vi "Begin.vi"(11 "Image Size":T1=enum."160x120") -> (0 "error out":errorcluster)   [LabVIEW 2012]
doc: "Called before other user functions, this VI is expected to open initial I/O refnums, load in file data, and do all program initialization. Notice that the <B>error out</B> terminal is simply used for data flow. Wiring it to other structures or subVIs ensures that this VI runs first."
uses:
  <vilib>/Rock Robotics/WPI/Camera/WPI_CameraImageSize.ctl
  <vilib>/Rock Robotics/WPI/Camera/WPI_CameraWhite Balance Values.ctl
  <vilib>/Rock Robotics/WPI/Camera/WPI_CameraExposure Values.ctl
  <vilib>/Rock Robotics/WPI/Camera/WPI_CameraFrameRate.ctl
  <vilib>/Rock Robotics/WPI/DriverStation/WPI_DriverStationRobotMode2.ctl
  <vilib>/Rock Robotics/SystemInterfaces/DIO/FPGA_DIOPWMChannel.ctl
  <vilib>/Rock Robotics/WPI/Joystick/WPI_JoystickDeviceEnum.ctl
  <vilib>/Rock Robotics/SystemInterfaces/Typedef/FPGA_TypedefDigitalModule.ctl
  Robot Global Data.vi
  <vilib>/Rock Robotics/WPI/MotorControl/WPI_MotorControlOpen Victor.vi
  <vilib>/Rock Robotics/SystemInterfaces/DIO/FPGA_DIOChannel.ctl
  <vilib>/Rock Robotics/SystemInterfaces/AI/FPGA_AIGyroChannel.ctl
  <vilib>/Rock Robotics/WPI/Relay/WPI_RelayDirection.ctl
  <vilib>/Rock Robotics/SystemInterfaces/DIO/FPGA_DIORelayChannel.ctl
  <vilib>/Rock Robotics/SystemInterfaces/AI/FPGA_AIChannel.ctl
  <vilib>/Rock Robotics/WPI/MotorControl/WPI_MotorControlOpen Jaguar.vi
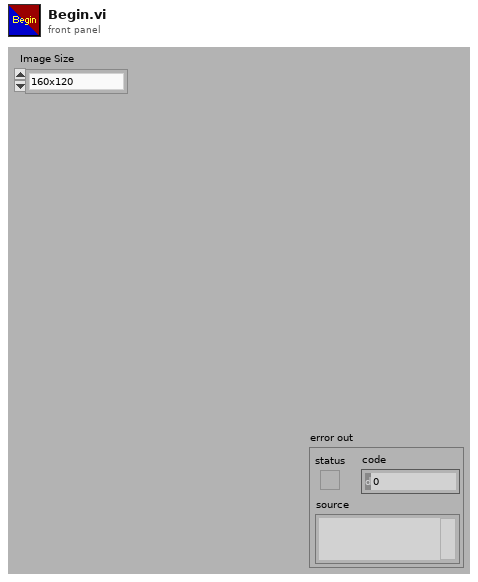
[diagram p1: front panel]
types:
  T1 = typedef "WPI_CameraImageSize.ctl" = enum16{"640x480", "320x240", "160x120"}
  T2 = typedef "FPGA_TypedefDigitalModule.ctl" = enum16{"Digital Module 1", "Digital Module 2"}
  T3 = typedef "FPGA_DIOPWMChannel.ctl" = enum8{"PWM 1", "PWM 2", "PWM 3", "PWM 4", "PWM 5", "PWM 6", "PWM 7", "PWM 8", "PWM 9", "PWM 10", "Invalid"}
  T4 = typedef "WPI_JoystickDeviceEnum.ctl" = enum16{"USB 1", "USB 2", "USB 3", "USB 4", "Kinect 1", "Kinect 2"}
  T5 = typedef "WPI_DriverStationRobotMode2.ctl" = enum16{"Autonomous Disabled", "Autonomous Enabled", "Teleop Disabled", "Teleop Enabled", "Timeout", "Finish", "Test Disabled", "Test Enabled"}
  T6 = typedef "WPI_CameraFrameRate.ctl" = u32
  T7 = typedef "WPI_CameraExposure Values.ctl" = enum16{"Auto", "Flicker-free 50 Hz", "Flicker-free 60 Hz", "Hold current"}
  T8 = typedef "WPI_CameraWhite Balance Values.ctl" = enum16{"Auto", "Fixed indoor", "Fixed outdoor 1", "Fixed outdoor 2", "Fixed fluorescent 1", "Fixed fluorescent 2", "Hold current"}
  T9 = typedef "WPI_CameraDevRef.ctl" = cluster{"Camera Address":string, "CameraStatus":errorcluster, "Acquire Image Notifier":refnum<notifier>}
  T10 = typedef "WPI_MotorControlDeviceRef.ctl" = cluster{"DeviceStatus":errorcluster, "Type":enum16{"PWM", "CAN"}, "PWM":cluster{"Digital Module":T2, "PWM Channel":T3, "DeadBand":T11}, "CAN":cluster{"Device Number":u8, "Control Mode":T12, "Semaphore":T13, "Max Vout":dbl}, "Invert":bool, "TransformRef":T14, "InvTransformRef":T14}
  T11 = typedef "WPI_PWMDeadband.ctl" = cluster{"Name":string, "maxPositivePwm":i32, "minPositivePwm":i32, "centerPwm":i32, "maxNegativePwm":i32, "minNegativePwm":i32, "angularRange":u16}
  T12 = typedef "WPI_CANJaguar_ControlMode.ctl" = enum8{"Percent VBus", "Current", "Speed", "Position", "Voltage"}
  T13 = typedef "Semaphore RefNum" = refnum<k1>
  T14 = typedef "WPI_PWMTransform_ConPane.ctl" = refnum<vi>
  T15 = typedef "WPI_JoystickDevRef.ctl" = cluster{"Device":T4}
  T16 = typedef "WPI_ServoDeviceRef.ctl" = cluster{"DeviceStatus":errorcluster, "Digital Module":T2, "PWM Channel":T3, "DeadBand":T11}
  T17 = typedef "FPGA_DIORelayChannel.ctl" = enum8{"Relay 1", "Relay 2", "Relay 3", "Relay 4", "Relay 5", "Relay 6", "Relay 7", "Relay 8", "Invalid"}
  T18 = typedef "WPI_RelayDirection.ctl" = enum16{"Both directions", "Forward only", "Reverse only"}
  T19 = typedef "WPI_RelayDevRef.ctl" = cluster{"DevStatus":errorcluster, "Relay Channel":T17, "Digital Module":T2, "Relay Direction":T18}
  T20 = typedef "FPGA_AIGyroChannel.ctl" = enum8{"AI 1", "AI 2", "Invalid"}
  T21 = typedef "FPGA_DIOChannel.ctl" = enum8{"DIO 1", "DIO 2", "DIO 3", "DIO 4", "DIO 5", "DIO 6", "DIO 7", "DIO 8", "DIO 9", "DIO 10", "DIO 11", "DIO 12", "DIO 13", "DIO 14", "Invalid"}
  T22 = typedef "FPGA_AIChannel.ctl" = enum8{"AI 1", "AI 2", "AI 3", "AI 4", "AI 5", "AI 6", "AI 7", "AI 8", "Invalid"}
  T23 = typedef "WPI_AnalogChannelDevRef.ctl" = cluster{"DevStatus":errorcluster, "Analog Module":T24, "Analog Channel":T22}
  T24 = typedef "FPGA_TypedefAnalogModule.ctl" = enum16{"Analog Module 1", "Analog Module 2"}
  T25 = typedef "WPI_DigitalInputDevRef.ctl" = cluster{"DevStatus":errorcluster, "DIO Channel":T21, "Digital Module":T2}
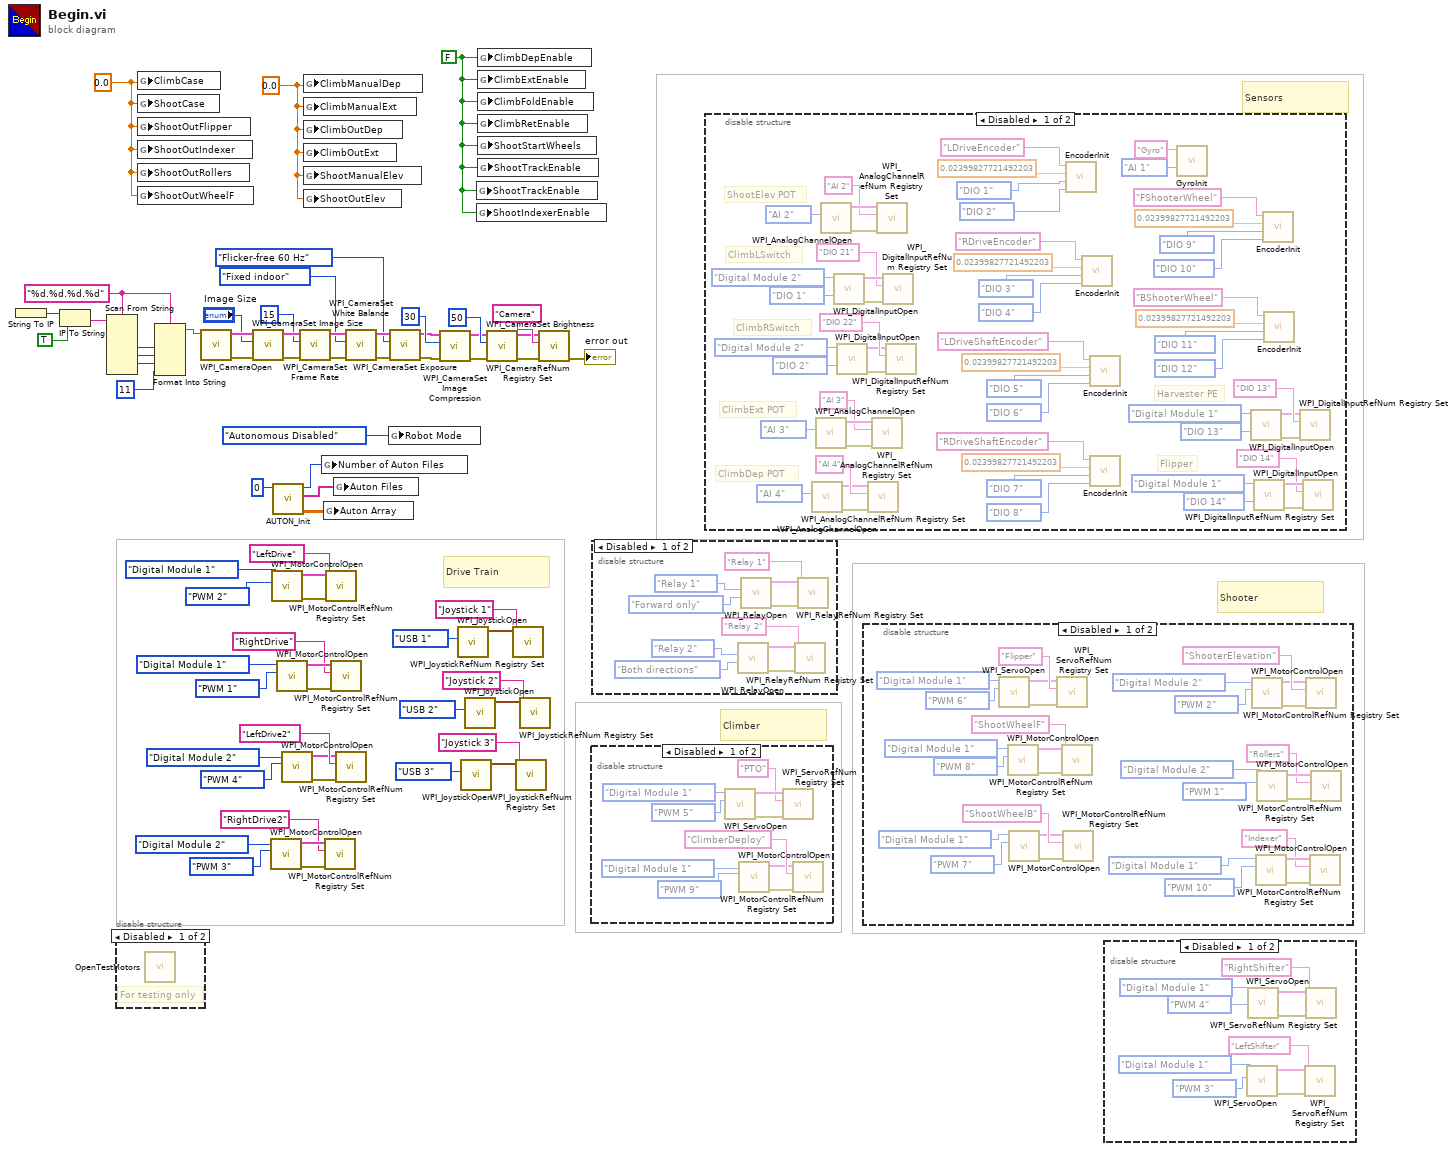
[diagram p0: block diagram]
diagram:
  w13 = FALSE ("ClimbDepEnable")
  w14 = 0.0 ("ClimbCase")
  w15 = 0.0 ("ClimbCase")
  w40 = "%d.%d.%d.%d" ("format string")
  # "Drive Train"
  # "Climber"
  # "Shooter"
  # "Sensors"
  n1 = String To IP() -> (0:w47:u32)  [unwired: 1 in]
  n2 = IP To String(1:TRUE ("dot notation? (F)"), 2:w47) -> (0:w45:string)
  n3 = Scan From String(format string=w40, input string=w45) -> (output 1=w44:i32, output 2=w43:i32, output 3=w42:i32)  [unwired: 7 in, 3 out]
  n4 = disable-structure shown="Disabled" {
    frame Disabled {
      # "For testing only"
      n5 = call "OpenTestMotors.vi"() -> ()  [unwired: 12 in]
    }
    frame Enabled {
    }
  }
  n6 = global write "Robot Global Data.vi" "ClimbCase"(w15) -> ()
  n7 = global write "Robot Global Data.vi" "ShootCase"(w15) -> ()
  n8 = global write "Robot Global Data.vi" "ShootOutFlipper"(w15) -> ()
  n9 = global write "Robot Global Data.vi" "ShootOutIndexer"(w15) -> ()
  n10 = global write "Robot Global Data.vi" "ShootOutRollers"(w15) -> ()
  n11 = global write "Robot Global Data.vi" "ShootOutWheelF"(w15) -> ()
  n12 = Format Into String(format string=w40, w44, w43, w42, 11 ("Compression")) -> (resulting string=w38:string)  [unwired: 2 in, 1 out]
  n13 = call <vilib>:"WPI_CameraOpen.vi"("Camera Address"=w38) -> ("error out"=w59:errorcluster, "CameraDevRef"=w60:T9)  [unwired: 1 in, 8 out]
  n14 = call <vilib>:"WPI_CameraSet Image Size.vi"("error in (no error)"=w59, "Image Size"="Image Size", "CameraDevRef"=w60) -> ("error out"=w58:errorcluster, "CameraDevRef Out"=w61:T9)  [unwired: 7 out]
  n15 = call-poly <vilib>:"WPI_MotorControlOpen.vi"("PWM Channel"=FPGA_DIOPWMChannel."PWM 3", "Digital Module (Module 1)"=FPGA_TypedefDigitalModule."Digital Module 2") -> ("error out"=w11:errorcluster, "MotorControlDeviceRef"=w10:T10)  [unwired: 8 in]
  n16 = call-poly <vilib>:"WPI_MotorControlOpen.vi"("PWM Channel"=FPGA_DIOPWMChannel."PWM 2", "Digital Module (Module 1)"=FPGA_TypedefDigitalModule."Digital Module 1") -> ("error out"=w25:errorcluster, "MotorControlDeviceRef"=w26:T10)  [unwired: 8 in]
  n17 = call "AUTON_Init.vi"("Default File"=0) -> ("Auton Array"=w33:dbl[][], "Auton Files"=w34:string[], "Number of Auton Files"=w35:i64)  [unwired: 8 in]
  n18 = call-poly <vilib>:"WPI_MotorControlOpen.vi"("PWM Channel"=FPGA_DIOPWMChannel."PWM 1", "Digital Module (Module 1)"=FPGA_TypedefDigitalModule."Digital Module 1") -> ("error out"=w32:errorcluster, "MotorControlDeviceRef"=w31:T10)  [unwired: 8 in]
  n19 = call-poly <vilib>:"WPI_MotorControlOpen.vi"("PWM Channel"=FPGA_DIOPWMChannel."PWM 4", "Digital Module (Module 1)"=FPGA_TypedefDigitalModule."Digital Module 2") -> ("error out"=w2:errorcluster, "MotorControlDeviceRef"=w3:T10)  [unwired: 8 in]
  n20 = call <vilib>:"WPI_CameraSet Frame Rate.vi"("error in (no error)"=w58, "Frame Rate (fps)"=T6 15, "CameraDevRef"=w61) -> ("error out"=w57:errorcluster, "CameraDevRef Out"=w63:T9)  [unwired: 7 out]
  n21 = global write "Robot Global Data.vi" "ClimbManualDep"(w14) -> ()
  n22 = global write "Robot Global Data.vi" "ClimbManualExt"(w14) -> ()
  n23 = global write "Robot Global Data.vi" "ClimbOutDep"(w14) -> ()
  n24 = global write "Robot Global Data.vi" "ClimbOutExt"(w14) -> ()
  n25 = global write "Robot Global Data.vi" "ShootManualElev"(w14) -> ()
  n26 = global write "Robot Global Data.vi" "ShootOutElev"(w14) -> ()
  n27 = global write "Robot Global Data.vi" "Number of Auton Files"(w35) -> ()
  n28 = global write "Robot Global Data.vi" "Auton Array"(w33) -> ()
  n29 = call <vilib>:"WPI_MotorControlRefNum Registry Set.vi"("error in (no error)"=w11, "refnum name"="RightDrive2", "MotorControlDevRef"=w10) -> ()  [unwired: 7 in, 2 out]
  n30 = call <vilib>:"WPI_MotorControlRefNum Registry Set.vi"("error in (no error)"=w25, "refnum name"="LeftDrive", "MotorControlDevRef"=w26) -> ()  [unwired: 7 in, 2 out]
  n31 = call <vilib>:"WPI_MotorControlRefNum Registry Set.vi"("error in (no error)"=w32, "refnum name"="RightDrive", "MotorControlDevRef"=w31) -> ()  [unwired: 7 in, 2 out]
  n32 = global write "Robot Global Data.vi" "Auton Files"(w34) -> ()
  n33 = call <vilib>:"WPI_MotorControlRefNum Registry Set.vi"("error in (no error)"=w2, "refnum name"="LeftDrive2", "MotorControlDevRef"=w3) -> ()  [unwired: 7 in, 2 out]
  n34 = call <vilib>:"WPI_CameraSet White Balance.vi"("error in (no error)"=w57, "White Balance"=WPI_CameraWhite_Balance_Values."Fixed indoor", "CameraDevRef"=w63) -> ("error out"=w56:errorcluster, "CameraDevRef Out"=w62:T9)  [unwired: 7 out]
  n35 = global write "Robot Global Data.vi" "Robot Mode"(WPI_DriverStationRobotMode2."Autonomous Disabled" ("Robot Mode")) -> ()
  n36 = call <vilib>:"WPI_CameraSet Exposure.vi"("error in (no error)"=w56, "Exposure"=WPI_CameraExposure_Values."Flicker-free 60 Hz", "CameraDevRef"=w62) -> ("error out"=w55:errorcluster, "CameraDevRef Out"=w65:T9)  [unwired: 7 out]
  n37 = call <vilib>:"WPI_CameraSet Image Compression.vi"("error in (no error)"=w55, "Compression"=30, "CameraDevRef"=w65) -> ("error out"=w54:errorcluster, "CameraDevRef Out"=w64:T9)  [unwired: 7 out]
  n38 = call <vilib>:"WPI_JoystickOpen.vi"("JoystickDevice"=WPI_JoystickDeviceEnum."USB 1") -> ("JoystickDevRef"=w16:T15)  [unwired: 10 in]
  n39 = call <vilib>:"WPI_JoystickOpen.vi"("JoystickDevice"=WPI_JoystickDeviceEnum."USB 3") -> ("JoystickDevRef"=w22:T15)  [unwired: 10 in]
  n40 = call <vilib>:"WPI_JoystickOpen.vi"("JoystickDevice"=WPI_JoystickDeviceEnum."USB 2") -> ("JoystickDevRef"=w21:T15)  [unwired: 10 in]
  n41 = global write "Robot Global Data.vi" "ShootTrackEnable"(w13) -> ()
  n42 = global write "Robot Global Data.vi" "ShootIndexerEnable"(w13) -> ()
  n43 = global write "Robot Global Data.vi" "ClimbDepEnable"(w13) -> ()
  n44 = global write "Robot Global Data.vi" "ClimbExtEnable"(w13) -> ()
  n45 = global write "Robot Global Data.vi" "ClimbFoldEnable"(w13) -> ()
  n46 = global write "Robot Global Data.vi" "ClimbRetEnable"(w13) -> ()
  n47 = global write "Robot Global Data.vi" "ShootStartWheels"(w13) -> ()
  n48 = global write "Robot Global Data.vi" "ShootTrackEnable"(w13) -> ()
  n49 = call <vilib>:"WPI_CameraSet Brightness.vi"("error in (no error)"=w54, "Brightness"=50, "CameraDevRef"=w64) -> ("error out"=w52:errorcluster, "CameraDevRef Out"=w53:T9)  [unwired: 7 out]
  n50 = call <vilib>:"WPI_JoystickRefNum Registry Set.vi"("refnum name"="Joystick 1", "JoystickDevRef"=w16) -> ()  [unwired: 8 in, 2 out]
  n51 = call <vilib>:"WPI_JoystickRefNum Registry Set.vi"("refnum name"="Joystick 3", "JoystickDevRef"=w22) -> ()  [unwired: 8 in, 2 out]
  n52 = call <vilib>:"WPI_JoystickRefNum Registry Set.vi"("refnum name"="Joystick 2", "JoystickDevRef"=w21) -> ()  [unwired: 8 in, 2 out]
  n53 = call <vilib>:"WPI_CameraRefNum Registry Set.vi"("error in (no error)"=w52, "refnum name"="Camera", "CameraDevRef"=w53) -> ("error out"=→"error out":errorcluster)  [unwired: 8 out]
  n54 = disable-structure shown="Disabled" {
    frame Disabled {
      n55 = call <vilib>:"WPI_ServoOpen.vi"("PWM Channel"=FPGA_DIOPWMChannel."PWM 5", "Digital Module (Module 1)"=FPGA_TypedefDigitalModule."Digital Module 1") -> ("error out"=w78:errorcluster, "ServoDeviceRef"=w77:T16)  [unwired: 8 in]
      n56 = call-poly <vilib>:"WPI_MotorControlOpen.vi"("PWM Channel"=FPGA_DIOPWMChannel."PWM 9", "Digital Module (Module 1)"=FPGA_TypedefDigitalModule."Digital Module 1") -> ("error out"=w72:errorcluster, "MotorControlDeviceRef"=w71:T10)  [unwired: 8 in]
      n57 = call <vilib>:"WPI_ServoRefNum Registry Set.vi"("error in (no error)"=w78, "refnum name"="PTO", "ServoDeviceRef"=w77) -> ()  [unwired: 7 in, 2 out]
      n58 = call <vilib>:"WPI_MotorControlRefNum Registry Set.vi"("error in (no error)"=w72, "refnum name"="ClimberDeploy", "MotorControlDevRef"=w71) -> ()  [unwired: 7 in, 2 out]
    }
    frame Enabled {
    }
  }
  n59 = disable-structure shown="Disabled" {
    frame Disabled {
      n60 = call <vilib>:"WPI_RelayOpen.vi"("Relay Direction"=WPI_RelayDirection."Both directions", "Relay Channel"=FPGA_DIORelayChannel."Relay 2") -> ("error out"=w79:errorcluster, "RelayDevRef"=w80:T19)  [unwired: 8 in]
      n61 = call <vilib>:"WPI_RelayOpen.vi"("Relay Direction"=WPI_RelayDirection."Forward only", "Relay Channel"=FPGA_DIORelayChannel."Relay 1") -> ("error out"=w88:errorcluster, "RelayDevRef"=w87:T19)  [unwired: 8 in]
      n62 = call <vilib>:"WPI_RelayRefNum Registry Set.vi"("error in (no error)"=w79, "refnum name"="Relay 2", "RelayDevRef"=w80) -> ()  [unwired: 7 in, 2 out]
      n63 = call <vilib>:"WPI_RelayRefNum Registry Set.vi"("error in (no error)"=w88, "refnum name"="Relay 1", "RelayDevRef"=w87) -> ()  [unwired: 7 in, 2 out]
    }
    frame Enabled {
    }
  }
  n64 = disable-structure shown="Disabled" {
    frame Disabled {
      # "ShootElev POT"
      # "ClimbRSwitch"
      # "ClimbLSwitch"
      # "ClimbDep POT"
      # "ClimbExt POT"
      # "Flipper"
      # "Harvester PE"
      n65 = call <vilib>:"WPI_AnalogChannelOpen.vi"("Analog Channel"=FPGA_AIChannel."AI 4") -> ("error out"=w113:errorcluster, "AIDeviceRef"=w114:T23)  [unwired: 9 in]
      n66 = call <vilib>:"WPI_AnalogChannelOpen.vi"("Analog Channel"=FPGA_AIChannel."AI 3") -> ("error out"=w112:errorcluster, "AIDeviceRef"=w111:T23)  [unwired: 9 in]
      n67 = call <vilib>:"WPI_AnalogChannelOpen.vi"("Analog Channel"=FPGA_AIChannel."AI 2") -> ("error out"=w95:errorcluster, "AIDeviceRef"=w97:T23)  [unwired: 9 in]
      n68 = call <vilib>:"WPI_DigitalInputOpen.vi"("DIO Channel"=FPGA_DIOChannel."DIO 1", "Digital Module (Module 1)"=FPGA_TypedefDigitalModule."Digital Module 2") -> ("error out"=w100:errorcluster, "DigitalInputDevRef"=w101:T25)  [unwired: 8 in]
      n69 = call <vilib>:"WPI_DigitalInputOpen.vi"("DIO Channel"=FPGA_DIOChannel."DIO 2", "Digital Module (Module 1)"=FPGA_TypedefDigitalModule."Digital Module 2") -> ("error out"=w107:errorcluster, "DigitalInputDevRef"=w106:T25)  [unwired: 8 in]
      n70 = call <vilib>:"WPI_AnalogChannelRefNum Registry Set.vi"("error in (no error)"=w113, "refnum name"="AI 4", "AIDeviceRef"=w114) -> ()  [unwired: 7 in, 2 out]
      n71 = call <vilib>:"WPI_AnalogChannelRefNum Registry Set.vi"("error in (no error)"=w112, "refnum name"="AI 3", "AIDeviceRef"=w111) -> ()  [unwired: 7 in, 2 out]
      n72 = call <vilib>:"WPI_AnalogChannelRefNum Registry Set.vi"("error in (no error)"=w95, "refnum name"="AI 2", "AIDeviceRef"=w97) -> ()  [unwired: 7 in, 2 out]
      n73 = call <vilib>:"WPI_DigitalInputRefNum Registry Set.vi"("error in (no error)"=w100, "refnum name"="DIO 21", "DigitalInputDevRef"=w101) -> ()  [unwired: 7 in, 2 out]
      n74 = call <vilib>:"WPI_DigitalInputRefNum Registry Set.vi"("error in (no error)"=w107, "refnum name"="DIO 22", "DigitalInputDevRef"=w106) -> ()  [unwired: 7 in, 2 out]
      n75 = call "EncoderInit.vi"("refnum name"="LDriveEncoder", "DistancePerCount"=0.02399827721492203, "DIO Channel"=FPGA_DIOChannel."DIO 1", "DIO Channel 2"=FPGA_DIOChannel."DIO 2") -> ()  [unwired: 7 in]
      n76 = call "EncoderInit.vi"("refnum name"="RDriveEncoder", "DistancePerCount"=0.02399827721492203, "DIO Channel"=FPGA_DIOChannel."DIO 3", "DIO Channel 2"=FPGA_DIOChannel."DIO 4") -> ()  [unwired: 7 in]
      n77 = call "EncoderInit.vi"("refnum name"="LDriveShaftEncoder", "DistancePerCount"=0.02399827721492203, "DIO Channel"=FPGA_DIOChannel."DIO 5", "DIO Channel 2"=FPGA_DIOChannel."DIO 6") -> ()  [unwired: 7 in]
      n78 = call "EncoderInit.vi"("refnum name"="RDriveShaftEncoder", "DistancePerCount"=0.02399827721492203, "DIO Channel"=FPGA_DIOChannel."DIO 7", "DIO Channel 2"=FPGA_DIOChannel."DIO 8") -> ()  [unwired: 7 in]
      n79 = call "GyroInit.vi"("refnum name"="Gyro", "Analog Channel"=FPGA_AIGyroChannel."AI 1") -> ()  [unwired: 8 in]
      n80 = call <vilib>:"WPI_DigitalInputOpen.vi"("DIO Channel"=FPGA_DIOChannel."DIO 13", "Digital Module (Module 1)"=FPGA_TypedefDigitalModule."Digital Module 1") -> ("error out"=w125:errorcluster, "DigitalInputDevRef"=w124:T25)  [unwired: 8 in]
      n81 = call <vilib>:"WPI_DigitalInputOpen.vi"("DIO Channel"=FPGA_DIOChannel."DIO 14", "Digital Module (Module 1)"=FPGA_TypedefDigitalModule."Digital Module 1") -> ("error out"=w118:errorcluster, "DigitalInputDevRef"=w119:T25)  [unwired: 8 in]
      n82 = call "EncoderInit.vi"("refnum name"="FShooterWheel", "DistancePerCount"=0.02399827721492203, "DIO Channel"=FPGA_DIOChannel."DIO 9", "DIO Channel 2"=FPGA_DIOChannel."DIO 10") -> ()  [unwired: 7 in]
      n83 = call "EncoderInit.vi"("refnum name"="BShooterWheel", "DistancePerCount"=0.02399827721492203, "DIO Channel"=FPGA_DIOChannel."DIO 11", "DIO Channel 2"=FPGA_DIOChannel."DIO 12") -> ()  [unwired: 7 in]
      n84 = call <vilib>:"WPI_DigitalInputRefNum Registry Set.vi"("error in (no error)"=w125, "refnum name"="DIO 13", "DigitalInputDevRef"=w124) -> ()  [unwired: 7 in, 2 out]
      n85 = call <vilib>:"WPI_DigitalInputRefNum Registry Set.vi"("error in (no error)"=w118, "refnum name"="DIO 14", "DigitalInputDevRef"=w119) -> ()  [unwired: 7 in, 2 out]
    }
    frame Enabled {
    }
  }
  n86 = disable-structure shown="Disabled" {
    frame Disabled {
      n87 = call <vilib>:"WPI_ServoOpen.vi"("PWM Channel"=FPGA_DIOPWMChannel."PWM 6", "Digital Module (Module 1)"=FPGA_TypedefDigitalModule."Digital Module 1") -> ("error out"=w152:errorcluster, "ServoDeviceRef"=w153:T16)  [unwired: 8 in]
      n88 = call-poly <vilib>:"WPI_MotorControlOpen.vi"("PWM Channel"=FPGA_DIOPWMChannel."PWM 8", "Digital Module (Module 1)"=FPGA_TypedefDigitalModule."Digital Module 1") -> ("error out"=w163:errorcluster, "MotorControlDeviceRef"=w164:T10)  [unwired: 8 in]
      n89 = call-poly <vilib>:"WPI_MotorControlOpen.vi"("PWM Channel"=FPGA_DIOPWMChannel."PWM 7", "Digital Module (Module 1)"=FPGA_TypedefDigitalModule."Digital Module 1") -> ("error out"=w149:errorcluster, "MotorControlDeviceRef"=w148:T10)  [unwired: 8 in]
      n90 = call <vilib>:"WPI_ServoRefNum Registry Set.vi"("error in (no error)"=w152, "refnum name"="Flipper", "ServoDeviceRef"=w153) -> ()  [unwired: 7 in, 2 out]
      n91 = call <vilib>:"WPI_MotorControlRefNum Registry Set.vi"("error in (no error)"=w163, "refnum name"="ShootWheelF", "MotorControlDevRef"=w164) -> ()  [unwired: 7 in, 2 out]
      n92 = call <vilib>:"WPI_MotorControlRefNum Registry Set.vi"("error in (no error)"=w149, "refnum name"="ShootWheelB", "MotorControlDevRef"=w148) -> ()  [unwired: 7 in, 2 out]
      n93 = call-poly <vilib>:"WPI_MotorControlOpen.vi"("PWM Channel"=FPGA_DIOPWMChannel."PWM 2", "Digital Module (Module 1)"=FPGA_TypedefDigitalModule."Digital Module 2") -> ("error out"=w174:errorcluster, "MotorControlDeviceRef"=w173:T10)  [unwired: 8 in]
      n94 = call-poly <vilib>:"WPI_MotorControlOpen.vi"("PWM Channel"=FPGA_DIOPWMChannel."PWM 10", "Digital Module (Module 1)"=FPGA_TypedefDigitalModule."Digital Module 1") -> ("error out"=w159:errorcluster, "MotorControlDeviceRef"=w160:T10)  [unwired: 8 in]
      n95 = call-poly <vilib>:"WPI_MotorControlOpen.vi"("PWM Channel"=FPGA_DIOPWMChannel."PWM 1", "Digital Module (Module 1)"=FPGA_TypedefDigitalModule."Digital Module 2") -> ("error out"=w169:errorcluster, "MotorControlDeviceRef"=w170:T10)  [unwired: 8 in]
      n96 = call <vilib>:"WPI_MotorControlRefNum Registry Set.vi"("error in (no error)"=w174, "refnum name"="ShooterElevation", "MotorControlDevRef"=w173) -> ()  [unwired: 7 in, 2 out]
      n97 = call <vilib>:"WPI_MotorControlRefNum Registry Set.vi"("error in (no error)"=w159, "refnum name"="Indexer", "MotorControlDevRef"=w160) -> ()  [unwired: 7 in, 2 out]
      n98 = call <vilib>:"WPI_MotorControlRefNum Registry Set.vi"("error in (no error)"=w169, "refnum name"="Rollers", "MotorControlDevRef"=w170) -> ()  [unwired: 7 in, 2 out]
    }
    frame Enabled {
    }
  }
  n99 = disable-structure shown="Disabled" {
    frame Disabled {
      n100 = call <vilib>:"WPI_ServoOpen.vi"("PWM Channel"=FPGA_DIOPWMChannel."PWM 3", "Digital Module (Module 1)"=FPGA_TypedefDigitalModule."Digital Module 1") -> ("error out"=w177:errorcluster, "ServoDeviceRef"=w184:T16)  [unwired: 8 in]
      n101 = call <vilib>:"WPI_ServoOpen.vi"("PWM Channel"=FPGA_DIOPWMChannel."PWM 4", "Digital Module (Module 1)"=FPGA_TypedefDigitalModule."Digital Module 1") -> ("error out"=w178:errorcluster, "ServoDeviceRef"=w179:T16)  [unwired: 8 in]
      n102 = call <vilib>:"WPI_ServoRefNum Registry Set.vi"("error in (no error)"=w177, "refnum name"="LeftShifter", "ServoDeviceRef"=w184) -> ()  [unwired: 7 in, 2 out]
      n103 = call <vilib>:"WPI_ServoRefNum Registry Set.vi"("error in (no error)"=w178, "refnum name"="RightShifter", "ServoDeviceRef"=w179) -> ()  [unwired: 7 in, 2 out]
    }
    frame Enabled {
    }
  }
